vi "Plot_symbol_to_tex.vi"(1 "Symbol array":u8[](array[numeric]), 2 "Legend":string[](array[string])) -> (0 "Tex String":string)   [LabVIEW 2010]
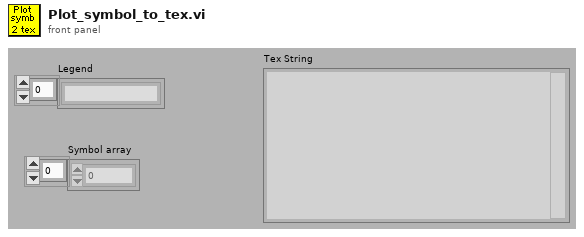
[diagram p1: front panel]
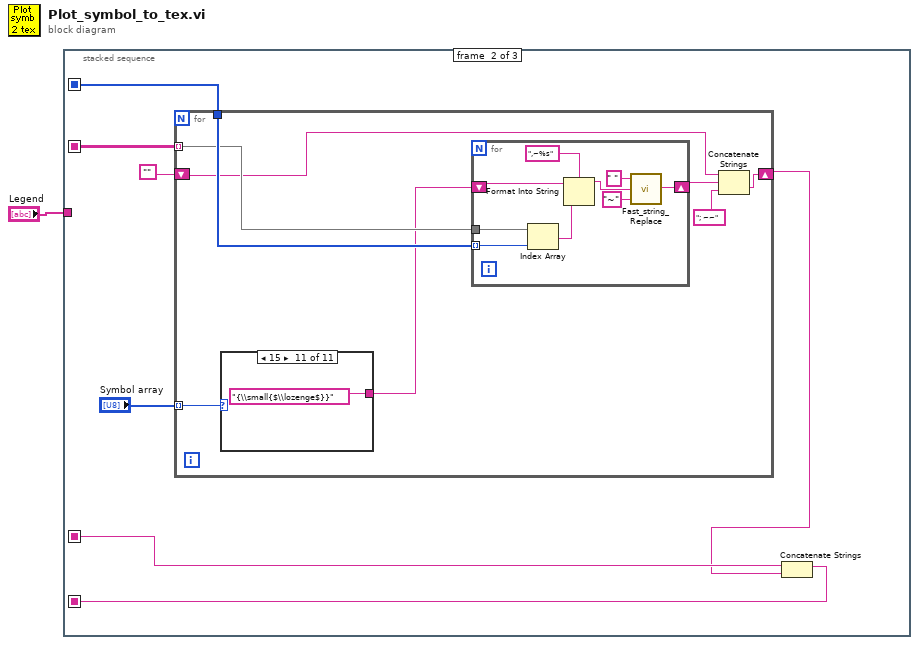
[diagram p0: block diagram]
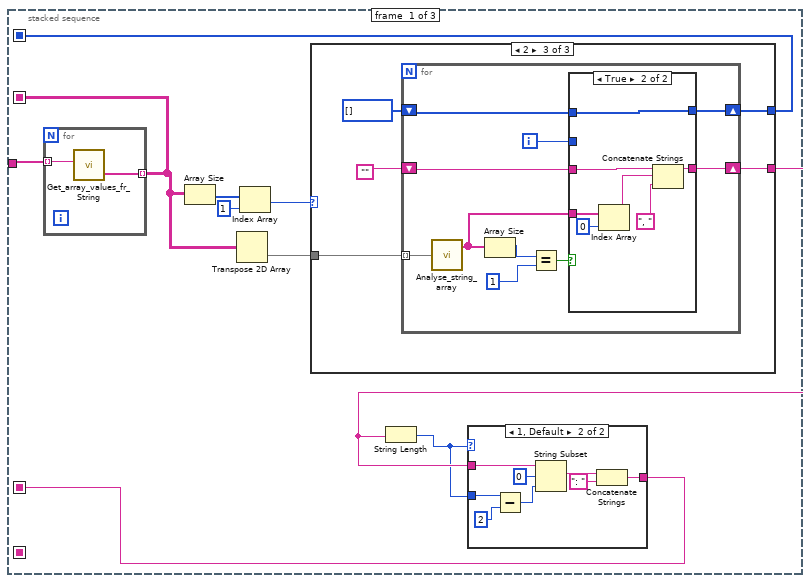
[diagram p2: hidden frame]
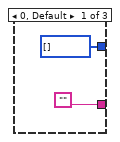
[diagram p4: hidden frame]
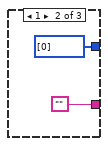
[diagram p5: hidden frame]
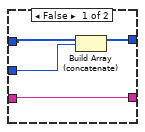
[diagram p6: hidden frame]
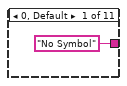
[diagram p7: hidden frame]
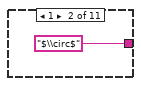
[diagram p8: hidden frame]
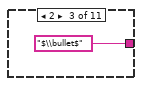
[diagram p9: hidden frame]
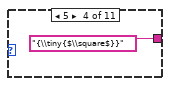
[diagram p10: hidden frame]
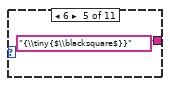
[diagram p11: hidden frame]
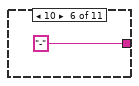
[diagram p12: hidden frame]
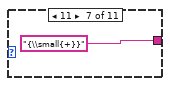
[diagram p13: hidden frame]
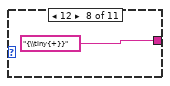
[diagram p14: hidden frame]
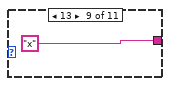
[diagram p15: hidden frame]
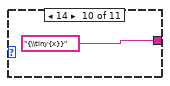
[diagram p16: hidden frame]
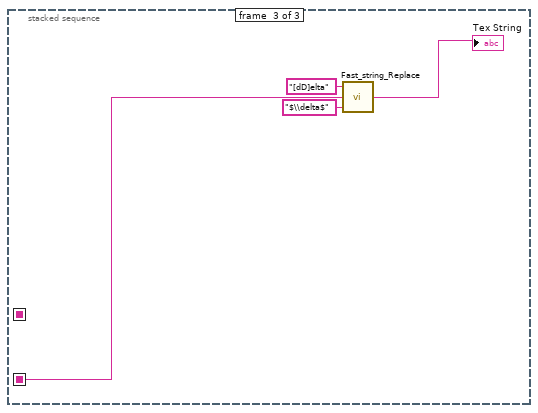
[diagram p17: hidden frame]
diagram:
  n1 = stacked-sequence {
    seq-local: [w7 _ _] -> [_ w58 _]
    seq-local: [w2 _ _] -> [_ w55 _]
    seq-local: [w6 _ _] -> [_ w57 _]
    seq-local: [_ w53 _] -> [_ _ w90]
    tunnel: "Legend" -> [w11 _ _]
    frame #0 {
      n2 = for {
        tunnel: w11 -> [w52] mode=indexing
        tunnel: [w51] -> w6 mode=indexing
        n3 = call "Get_array_values_fr_String.vi"("String Value"=w52) -> ("String array"=w51:string[])  [unwired: 1 out]
      }
      n4 = Array Size(array=w6) -> (size(s)=w10:i32[])
      n5 = Transpose 2D Array(2D array=w6) -> (transposed array=w8:string[][])
      n6 = Index Array(array=w10, index=1) -> (element=w5:i32)
      n7 = case shown="2" w5 {
        tunnel: w8 -> [_ _ w29]
        tunnel: [i32[] [] i32[] [0] w27] -> w7
        tunnel: ["" "" w26] -> w4
        frame 0, Default {
        }
        frame 1 {
        }
        frame 2 {
          n8 = for {
            tunnel: w29 -> [w39] mode=indexing
            shift-right: [w33] -> w26
            shift-left: "" -> [w34]
            shift-right: [w31] -> w27
            shift-left: i32[] [] -> [w32]
            i -> [w30]
            n9 = call "Analyse_string_array.vi"("String array"=w39) -> ("Unique strings"=w35:string[])  [unwired: 1 in, 1 out]
            n10 = Array Size(array=w35) -> (size(s)=w38:i32)
            n11 = Equal?(x=w38, y=1) -> (x = y?=w36:bool)
            n12 = case shown="True" w36 {
              tunnel: w35 -> [_ w50]
              tunnel: w34 -> [w40 w47]
              tunnel: [w40 w46] -> w33
              tunnel: w32 -> [w42 w45]
              tunnel: [w41 w45] -> w31
              tunnel: w30 -> [w43 _]
              frame False {
                n13 = Build Array (concatenate)(w42, w43) -> (w41:i32[])
              }
              frame True {
                n14 = Index Array(array=w50, index=0) -> (element=w48:string)
                n15 = Concatenate Strings(w47, w48, ", " ("string")) -> (w46:string)
              }
            }
          }
        }
      }
      n16 = String Length(string=w4) -> (length=w3:i32)
      n17 = case shown="1, Default" w3 {
        tunnel: w4 -> [w12 w19]
        tunnel: w3 -> [_ w15]
        tunnel: [w12 w16] -> w2
        frame 0 {
        }
        frame 1, Default {
          n18 = Subtract(x=w15, y=2) -> (x-y=w14:i32)
          n19 = String Subset(string=w19, offset (0)=0, length (rest)=w14) -> (substring=w18:string)
          n20 = Concatenate Strings(w18, ": " ("string")) -> (w16:string)
        }
      }
    }
    frame #1 {
      n21 = for {
        tunnel: "Symbol array" -> [w67] mode=indexing
        tunnel: w58 -> [w66]
        tunnel: w57 -> [w65] mode=indexing
        shift-right: [w63] -> w54
        shift-left: "" -> [w60]
        n22 = case shown="15" w67 {
          tunnel: ["No Symbol" "$\\circ$" "$\\bullet$" "{\\tiny{$\\square$}}" "{\\tiny{$\\blacksquare$}}" "-" "{\\small{+}}" "{\\tiny{+}}" "x" "{\\tiny{x}}" "{\\small{$\\lozenge$}}"] -> w61
          frame 0, Default {
          }
          frame 1 {
          }
          frame 2 {
          }
          frame 5 {
          }
          frame 6 {
          }
          frame 10 {
          }
          frame 11 {
          }
          frame 12 {
          }
          frame 13 {
          }
          frame 14 {
          }
          frame 15 {
          }
        }
        n23 = for {
          tunnel: w66 -> [w76] mode=indexing
          tunnel: w65 -> [w75]
          shift-right: [w70] -> w64
          shift-left: w61 -> [w74]
          n24 = Index Array(array=w75, index=w76) -> (element=w73:string)
          n25 = Format Into String(format string=",~%s", initial string=w74, w73) -> (resulting string=w71:string)  [unwired: 1 in, 1 out]
          n26 = call "Fast_string_Replace.vi"("Replace match with:"="~", "Input String"=w71, "regular expression"=" ") -> ("Output String"=w70:string)  [unwired: 1 in, 1 out]
        }
        n27 = Concatenate Strings(w60, w64, "; ~~" ("string")) -> (w63:string)
      }
      n28 = Concatenate Strings(w55, w54) -> (w53:string)
    }
    frame #2 {
      n29 = call "Fast_string_Replace.vi"("Replace match with:"="$\\delta$", "Input String"=w90, "regular expression"="[dD]elta") -> ("Output String"=→"Tex String":string)  [unwired: 1 in, 1 out]
    }
  }
